vi "TimingLoop.vi"(8 "Error In":errorcluster, 11 "Message Queues":T1) -> (0 "Error Out":errorcluster)   [LabVIEW 2017, in "Server.lvlib" / "Timing.lvlib"]
doc: "This Loop is responsible for sending cyclic messages to MHL."
uses:
  Timing.lvlib
  Message Queue/CommReferences.ctl
  Message Queue/MessageCluster.ctl
  MessageSetList.ctl
  MessageSet.ctl
  <vilib>/Utility/error.llb/Error Cluster From Error Code.vi
  Message Queue/EnqueueMessage(Single).vi
  <vilib>/ErrorRing/Error Ring.xnode
  Message Queue/Message Queue.lvlib
  ErrorLogger/ErrorLogger.lvlib
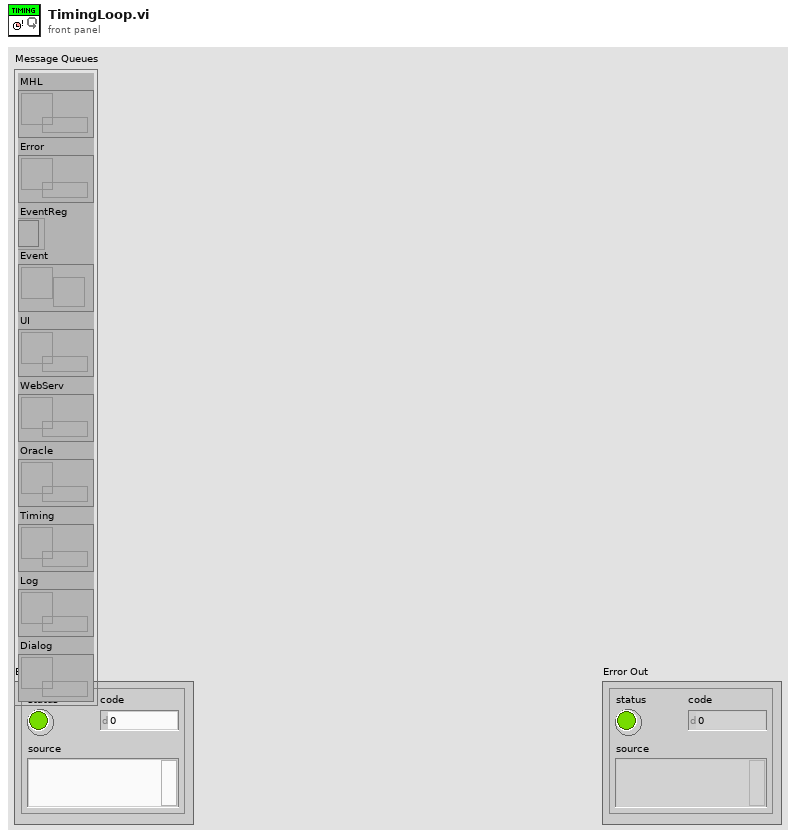
[diagram p1: front panel]
types:
  T1 = typedef "Server.lvlib/Message Queue.lvlib/CommReferences.ctl" = cluster{"MHL":refnum<queue>, "Error":refnum<queue>, "EventReg":refnum<event-registration>, "Event":refnum<user-event>, "UI":refnum<queue>, "WebServ":refnum<queue>, "Oracle":refnum<queue>, "Timing":refnum<queue>, "Log":refnum<queue>, "Dialog":refnum<queue>}
  T2 = typedef "Server.lvlib/Timing.lvlib/MessageSetList.ctl" = T3[]
  T3 = typedef "Server.lvlib/Timing.lvlib/MessageSet.ctl" = cluster{"MessageName":string, "Frequency (s)":dbl, "LastTime":timestamp}
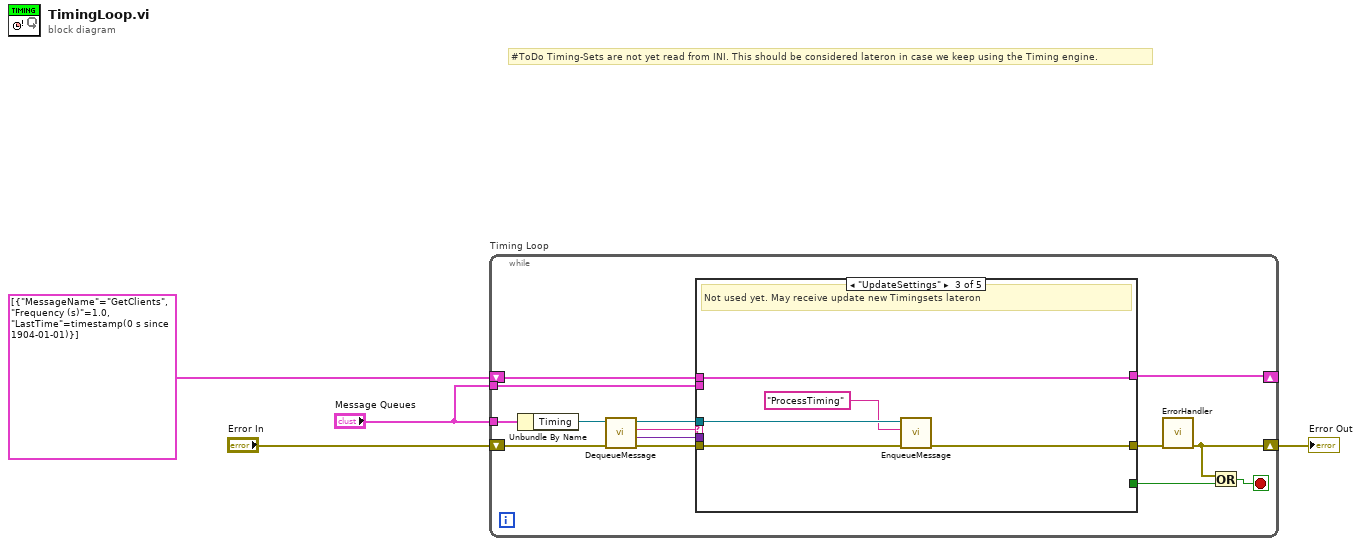
[diagram p0: block diagram]
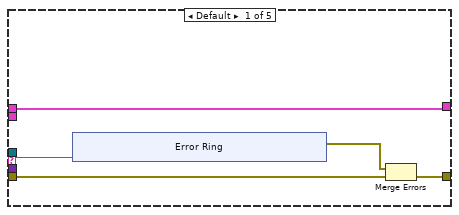
[diagram p2: hidden frame]
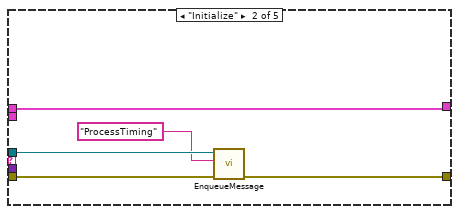
[diagram p3: hidden frame]
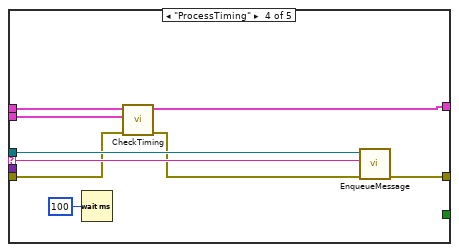
[diagram p4: hidden frame]
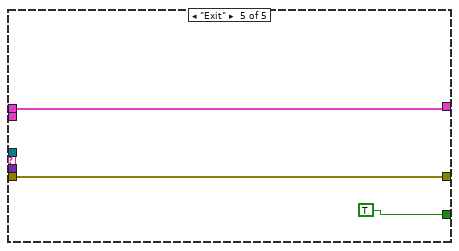
[diagram p5: hidden frame]
diagram:
  # "#ToDo Timing-Sets are not yet read from INI. This should be considered lateron in case we keep using the Timing engine."
  n1 = while "Timing Loop" {
    shift-right: [w5] -> w3
    shift-left: "Error In" -> [w18]
    tunnel: "Message Queues" -> [w13]
    shift-right: [w14] -> _
    shift-left: T2 [{"MessageName"="GetClients", "Frequency (s)"=1.0, "LastTime"=timestamp(0 s since 1904-01-01)}] -> [w15]
    tunnel: "Message Queues" -> [w7]
    stop <- w6 stop-if-true
    n2 = Unbundle By Name(w13) -> ("Timing"=w12:refnum<queue>)
    n3 = call "DequeueMessage.vi"("error in (no error)"=w18, "Message Queue"=w12) -> ("error out"=w16:errorcluster, "Message Data"=w10:variant, "Message"=w11:string, "dup Message Queue"=w9:refnum<queue>)  [unwired: 5 in, 1 out]
    n4 = case shown="\"UpdateSettings\"" w11 {
      selector: w11 -> [w21 _ _ w47 _]
      tunnel: [w20 w33 w38 w49 w52] -> w17
      tunnel: w16 -> [w23 w35 w40 w43 w52]
      tunnel: [w22 w34 w39 w45 w51] -> w14
      tunnel: w15 -> [w22 w34 w39 w46 w51]
      tunnel: w10 -> [_ _ _ _ _]
      tunnel: w9 -> [_ w32 w37 w48 _]
      tunnel: [_ _ _ _ TRUE] -> w8
      tunnel: w7 -> [_ _ _ w42 _]
      frame Default {
        n5 = xnode "Error Ring"("parameter 0"=w21) -> ("error out"=w19:errorcluster)
        n6 = Merge Errors(w19, w23) -> (w20:errorcluster)
      }
      frame "Initialize" {
        n7 = call-poly "EnqueueMessage.vi"("error in (no error)"=w35, "Message"="ProcessTiming", "Message Queue"=w32) -> ("error out"=w33:errorcluster)  [unwired: 7 in, 1 out]
      }
      frame "UpdateSettings" {
        # "Not used yet. May receive update new Timingsets lateron"
        n8 = call-poly "EnqueueMessage.vi"("error in (no error)"=w40, "Message"="ProcessTiming", "Message Queue"=w37) -> ("error out"=w38:errorcluster)  [unwired: 7 in, 1 out]
      }
      frame "ProcessTiming" {
        n9 = Wait (ms)(milliseconds to wait=u32 100) -> ()  [unwired: 1 out]
        n10 = call "CheckTiming.vi"("error in (no error)"=w43, "Message Queues"=w42, "MessageSetList"=w46) -> ("error out"=w41:errorcluster, "Array"=w45:T3[])  [unwired: 7 in]
        n11 = call-poly "EnqueueMessage.vi"("error in (no error)"=w41, "Message"=w47, "Message Queue"=w48) -> ("error out"=w49:errorcluster)  [unwired: 7 in, 1 out]
      }
      frame "Exit" {
      }
    }
    n12 = call "ErrorHandler.vi"("error in (no error)"=w17) -> ("error out"=w5:errorcluster)  [unwired: 10 in]
    n13 = Or(x=w5, y=w8) -> (x .or. y?=w6:bool)
  }
  "Error Out" <- w3
